vi "TMCM351-getSpeed.vi"(4 "错误输入":errorcluster caption="错误输入（无错误）", 7 "com in":refnum<visa-resource-name>) -> (0 "错误输出":errorcluster, 1 "Motion Done":bool, 2 "speed out":i32[](array[numeric]), 3 "com out":refnum<visa-resource-name>)   [LabVIEW 2018]
uses:
  module_param.vi
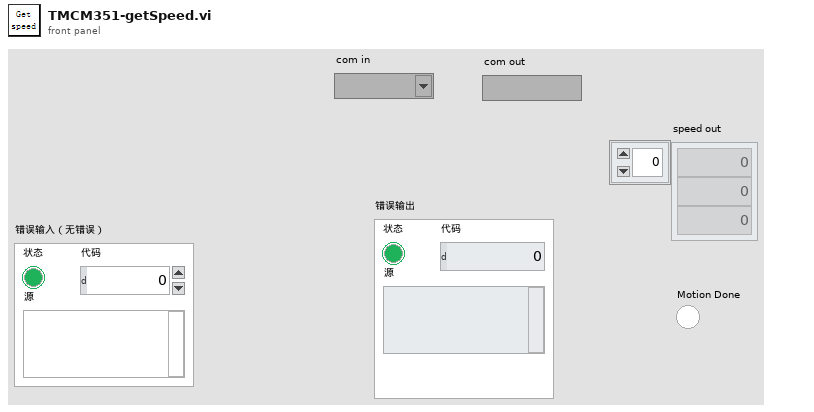
[diagram p1: front panel]
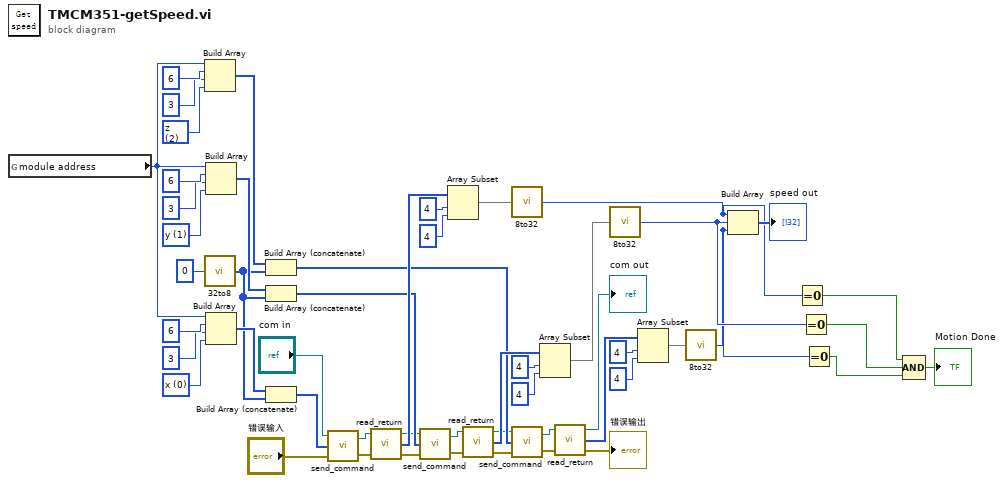
[diagram p0: block diagram]
diagram:
  w12 = u8 2 items=["x", "y", "z"] ("motor")
  w26 = u8 0 items=["x", "y", "z"] ("motor")
  w37 = u8 1 items=["x", "y", "z"] ("motor")
  n1 = global read "module_param.vi" "module address"() -> (w13:u8)
  n2 = Build Array(w13, u8 6, u8 3, w12) -> (w23:u8[])
  n3 = call "32to8.vi"("32data_in"=0) -> ("8Array"=w8:u8[])
  n4 = Build Array(w13, u8 6, u8 3, w37) -> (w36:u8[])
  n5 = Build Array(w13, u8 6, u8 3, w26) -> (w50:u8[])
  n6 = Build Array (concatenate)(w23, w8) -> (w22:u8[])
  n7 = Build Array (concatenate)(w36, w8) -> (w35:u8[])
  n8 = Build Array (concatenate)(w50, w8) -> (w49:u8[])
  n9 = call "send_command.vi"("错误输入"="错误输入", 3:w49, "com in"="com in") -> ("错误输出"=w46:errorcluster, "com out"=w47:refnum<visa-resource-name>)
  n10 = call "read_return.vi"("错误输入（无错误）"=w46, "com in"=w47) -> ("错误输出"=w33:errorcluster, "return out"=w44:u8[], "com out"=w34:refnum<visa-resource-name>)  [unwired: 1 in]
  n11 = call "send_command.vi"("错误输入"=w33, 3:w35, "com in"=w34) -> ("错误输出"=w31:errorcluster, "com out"=w32:refnum<visa-resource-name>)
  n12 = Array Subset(array=w44, index=4 ("索引"), length=4 ("长度")) -> (w41:u8[])
  n13 = call "read_return.vi"("错误输入（无错误）"=w31, "com in"=w32) -> ("错误输出"=w14:errorcluster, "return out"=w27:u8[], "com out"=w15:refnum<visa-resource-name>)  [unwired: 1 in]
  n14 = call "8to32.vi"("Arrayin"=w41) -> ("data32"=w7:i32)
  n15 = call "send_command.vi"("错误输入"=w14, 3:w22, "com in"=w15) -> ("错误输出"=w20:errorcluster, "com out"=w21:refnum<visa-resource-name>)
  n16 = Array Subset(array=w27, index=4 ("索引"), length=4 ("长度")) -> (w28:u8[])
  n17 = call "read_return.vi"("错误输入（无错误）"=w20, "com in"=w21) -> ("错误输出"=→"错误输出":errorcluster, "return out"=w16:u8[], "com out"=→"com out":refnum<visa-resource-name>)  [unwired: 1 in]
  n18 = call "8to32.vi"("Arrayin"=w28) -> ("data32"=w6:i32)
  n19 = Array Subset(array=w16, index=4 ("索引"), length=4 ("长度")) -> (w17:u8[])
  n20 = call "8to32.vi"("Arrayin"=w17) -> ("data32"=w5:i32)
  n21 = Build Array(w7, w6, w5) -> (→"speed out":i32[])
  n22 = Equal To 0?(x=w7) -> (x = 0?=w4:bool)
  n23 = Equal To 0?(x=w6) -> (x = 0?=w3:bool)
  n24 = Equal To 0?(x=w5) -> (x = 0?=w2:bool)
  n25 = Compound Arithmetic op=AND ("复合运算")(w4, w3, w2) -> (→"Motion Done":bool)
